vi "TextWithValueArray.vi"(5 "Group":string, 6 "Headers":string[](array[string]), 7 "Values":dbl[](array[numeric]), 9 "Origin":cluster{"X":i32, "Y":i32}, 10 "Font Size":i16=20, 11 "Image in":T1) -> (3 "Image out":T1)   [LabVIEW 2015]
uses:
  <vilib>/vision/Image Controls.llb/IMAQ Image.ctl
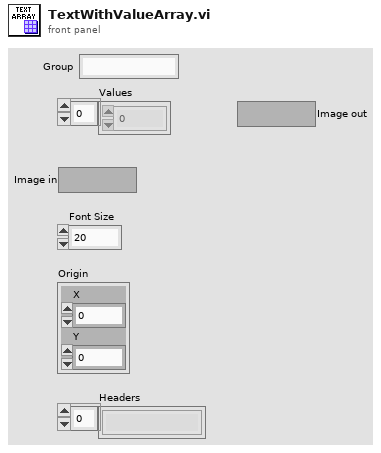
[diagram p1: front panel]
types:
  T1 = typedef "IMAQ Image.ctl" = refnum<image>
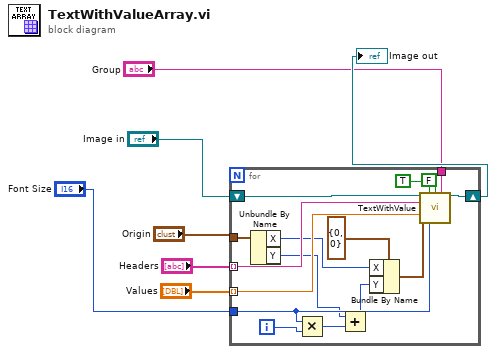
[diagram p0: block diagram]
diagram:
  n1 = for {
    tunnel: "Origin" -> [w15]
    tunnel: "Headers" -> [w21] mode=indexing
    shift-right: [w23] -> w5
    shift-left: "Image in" -> [w22]
    tunnel: "Values" -> [w20] mode=indexing
    tunnel: "Font Size" -> [w12]
    tunnel: "Group" -> [w8]
    i -> [w13]
    n2 = Unbundle By Name(w15) -> ("X"=w14:i32, "Y"=w9:i32)
    n3 = Multiply(x=w12, y=w13) -> (x*y=w11:i32)
    n4 = Add(x=w9, y=w11) -> (x+y=w10:i32)
    n5 = Bundle By Name(cluster=cluster{"X":i32, "Y":i32} {"X"=0, "Y"=0} ("Origin"), "X"=w14, "Y"=w10) -> (w16:cluster{"X":i32, "Y":i32})
    n6 = call "TextWithValue.vi"("Refnum in"=w22, "Visible"=TRUE, "IsError"=FALSE, "Group"=w8, "Header"=w21, "Value"=w20, "Origin"=w16, "[User-specified Font].Size"=w12) -> ("Refnum out"=w23:T1)  [unwired: 7 in]
  }
  "Image out" <- w5
